vi "Initialise.vi"(8 "error in (no error)":errorcluster, 11 "LSM9DS1 IMU in":refnum<class "LSM9DS1 IMU.lvclass">) -> (0 "error out":errorcluster, 3 "LSM9DS1 IMU out":refnum<class "LSM9DS1 IMU.lvclass">)   [LabVIEW 2020, in "LSM9DS1 IMU.lvclass"]
doc: "Initialises the IMU with basic default values."
uses:
  LSM9DS1 IMU.lvclass
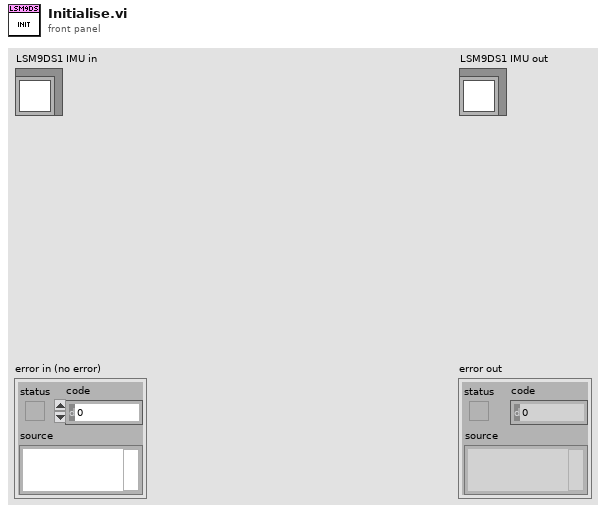
[diagram p1: front panel]
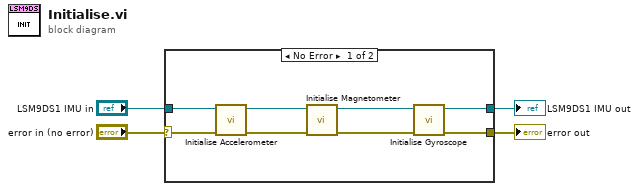
[diagram p0: block diagram]
diagram:
  n1 = case shown="No Error" "error in (no error)" {
    selector: "error in (no error)" -> [w6 w14]
    tunnel: [w5 w14] -> w3
    tunnel: [w9 w13] -> w1
    tunnel: "LSM9DS1 IMU in" -> [w12 w13]
    frame No Error {
      n2 = call "Initialise Accelerometer.vi"("error in (no error)"=w6, "LSM9DS1 IMU in"=w12) -> ("error out"=w7:errorcluster, "LSM9DS1 IMU out"=w11:refnum<class "LSM9DS1 IMU.lvclass">)  [unwired: 8 in]
      n3 = call "Initialise Magnetometer.vi"("error in (no error)"=w7, "LSM9DS1 IMU in"=w11) -> ("error out"=w8:errorcluster, "LSM9DS1 IMU out"=w10:refnum<class "LSM9DS1 IMU.lvclass">)  [unwired: 8 in]
      n4 = call "Initialise Gyroscope.vi"("error in (no error)"=w8, "LSM9DS1 IMU in"=w10) -> ("error out"=w5:errorcluster, "LSM9DS1 IMU out"=w9:refnum<class "LSM9DS1 IMU.lvclass">)  [unwired: 8 in]
    }
    frame Error {
    }
  }
  "error out" <- w3
  "LSM9DS1 IMU out" <- w1
